vi "Operation Stop.vi"(8 "error in (no error)":errorcluster, 11 "Superior Actor in":refnum<class "Root Actor.lvclass">) -> (0 "error out":errorcluster, 3 "Superior Actor out":refnum<class "Root Actor.lvclass">)   [LabVIEW 2024, in "Root Actor.lvclass"]
uses:
  Root Actor.lvclass
  C:/Users/iio/Desktop/Bussiness/Tricorn Re/Madelbrot 4.0/General Library/Ancestor Class/Actor/System Actor/System Actor.lvclass
  Root Actor.lvclass/Root Actor.ctl
  Public Data/Read Node Controller.vi
  Actor Assistant/Root Actor Node Controller/Node Controller.lvclass
  Messenger/Messenger/Messenger.lvclass
  Notifier Controller/Notifier Controller.lvclass
  Circular Buffer/Circular Buffer.lvclass
  System Actor/System Actor.lvclass
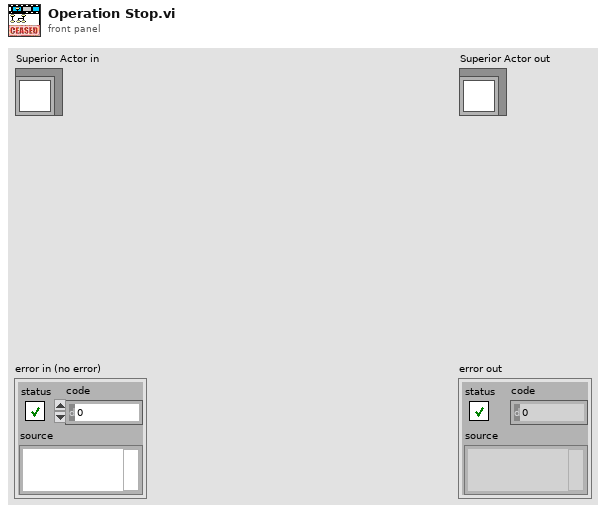
[diagram p1: front panel]
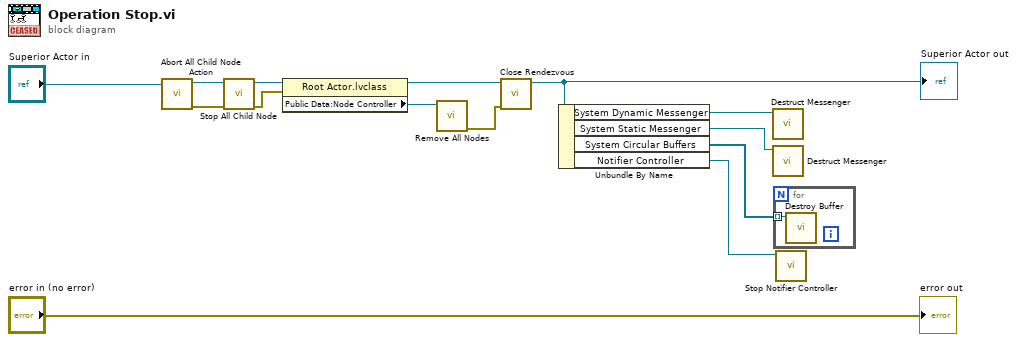
[diagram p0: block diagram]
diagram:
  n1 = call "Abort All Child Node Action.vi"("Root Actor in"="Superior Actor in") -> ("error out"=w8:errorcluster, "Root Actor out"=w11:refnum<class "Root Actor.lvclass">)  [unwired: 9 in]
  n2 = call-dynamic "Stop All Child Node.vi"("error in (no error)"=w8, "Root Actor in"=w11) -> ("error out"=w7:errorcluster, "Root Actor out"=w10:refnum<class "Root Actor.lvclass">)  [unwired: 8 in]
  n3 = property class="Root Actor.lvclass"(reference=w10, error in=w7) -> (reference out=w6:refnum<class "Root Actor.lvclass">, "Public Data:Node Controller"=w9:refnum<class "Node Controller.lvclass">)  [unwired: 1 out]
  n4 = call-dynamic "Remove All Nodes.vi"("Node Controller in"=w9) -> ("error out"=w5:errorcluster)  [unwired: 9 in, 1 out]
  n5 = call "Close Rendezvous.vi"("error in (no error)"=w5, "System Actor in"=w6) -> ("System Actor out"=w13:refnum<class "Root Actor.lvclass">)  [unwired: 8 in, 1 out]
  "Superior Actor out" <- w13
  n6 = Unbundle By Name(w13) -> ("System Dynamic Messenger"=w1:refnum<class "Messenger.lvclass">, "System Static Messenger"=w4:refnum<class "Messenger.lvclass">, "System Circular Buffers"=w3:refnum<class "Circular Buffer.lvclass">[], "Notifier Controller"=w2:refnum<class "Notifier Controller.lvclass">)
  n7 = call-dynamic "Destruct Messenger.vi"("Messenger Component in"=w1) -> ()  [unwired: 9 in, 2 out]
  n8 = call-dynamic "Destruct Messenger.vi"("Messenger Component in"=w4) -> ()  [unwired: 9 in, 2 out]
  n9 = for {
    tunnel: w3 -> [w15] mode=indexing
    n10 = call-dynamic "Destroy Buffer.vi"("Circular Buffer in"=w15) -> ()  [unwired: 9 in, 2 out]
  }
  n11 = call-dynamic "Stop Notifier Controller.vi"("Notifier Controller in"=w2) -> ()  [unwired: 9 in, 2 out]
  "error out" <- "error in (no error)"
